vi "VCS Read Channel Data Vector.vi"(0 "axis in":cluster{"keyHandle":u32, "nodeId":u16}={"keyHandle"=0, "nodeId"=1}, 5 "channelNumber":u8, 7 "vectorSize":u32, 9 "objectSize":u8, 11 "error in (no error)":errorcluster) -> (4 "axis out":cluster{"keyHandle":u32, "nodeId":u16}={"keyHandle"=0, "nodeId"=1}, 8 "data vector":u8[](array[numeric]), 15 "error out":errorcluster)   [LabVIEW 2018]
doc: "<B>VCS_ReadChannelDataVector</B> returns the data points of a selected channel."
uses:
  Resources/EposCmd.dll
  Resources/EposCmd64.dll
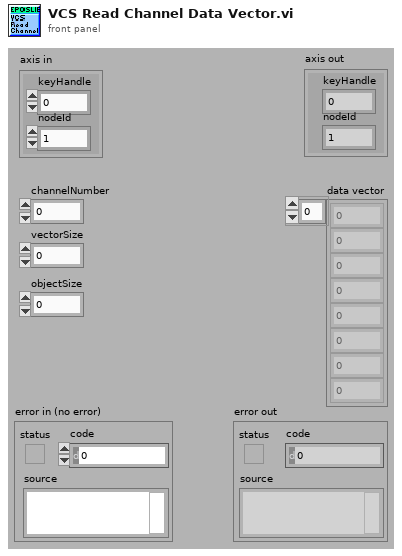
[diagram p1: front panel]
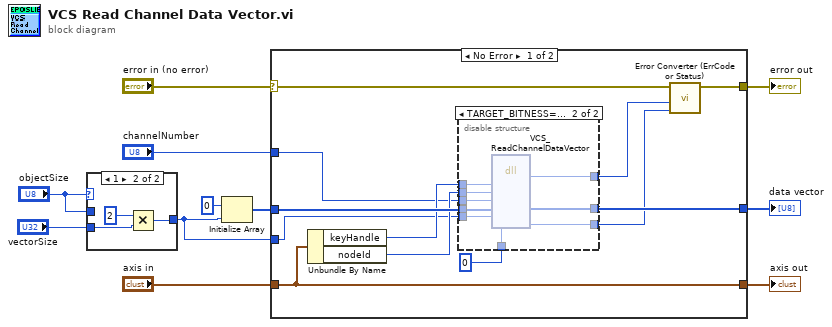
[diagram p0: block diagram]
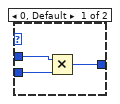
[diagram p2: hidden frame]
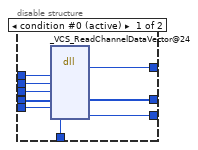
[diagram p3: hidden frame]
diagram:
  n1 = case shown="1" "objectSize" {
    tunnel: "vectorSize" -> [w13 w17]
    tunnel: "objectSize" -> [w14 _]
    tunnel: [w12 w15] -> w1
    frame 0, Default {
      n2 = Multiply(x=w14, y=w13) -> (x*y=w12:u32)
    }
    frame 1 {
      n3 = Multiply(x=u32 2, y=w17) -> (x*y=w15:u32)
    }
  }
  n4 = Initialize Array(u8 0, w1) -> (w6:u8[])
  n5 = case shown="No Error" "error in (no error)" {
    selector: "error in (no error)" -> [w27 w49]
    tunnel: "axis in" -> [w29 w50]
    tunnel: [w29 w50] -> w10
    tunnel: [w28 w49] -> w9
    tunnel: w6 -> [w26 w48]
    tunnel: [w25 w48] -> w5
    tunnel: "channelNumber" -> [w22 _]
    tunnel: w1 -> [w18 _]
    frame No Error {
      n6 = Unbundle By Name(w29) -> ("keyHandle"=w24:u32, "nodeId"=w23:u16)
      n7 = disable-structure shown="TARGET_BITNESS==64" {
        disable-tunnel: w26 -> [w38 w47]
        disable-tunnel: [w37 w46] -> w25
        disable-tunnel: w24 -> [w36 w45]
        disable-tunnel: w23 -> [w35 w44]
        disable-tunnel: w22 -> [w34 w43]
        disable-tunnel: u32 0 ("pErrorCode") -> [w33 w42]
        disable-tunnel: [w32 w41] -> w20
        disable-tunnel: [w31 w40] -> w19
        disable-tunnel: w18 -> [w30 w39]
        frame condition #0 (active) {
          n8 = dll-call lib="C:/Projeto em LabVIEW/EPOS-LabVIEW-Instrument-Driver-En/LabVIEW/maxon EPOS/Resources/EposCmd.*" fn="_VCS_ReadChannelDataVector@24" ("VCS_ReadChannelDataVector")("KeyHandle"=w36, "NodeId"=w35, "ChannelNumber"=w34, "pDataVector"=w38, "VectorSize"=w30, "pErrorCode"=w33) -> ("Rückgabetyp"=w31:i32, "pDataVector"=w37:u8[], "pErrorCode"=w32:u32)  [unwired: 7 in, 2 out]
        }
        frame condition #1 {
          n9 = dll-call lib="C:/setup/Resources/EposCmd64.*" fn="VCS_ReadChannelDataVector"("KeyHandle"=w45, "NodeId"=w44, "ChannelNumber"=w43, "pDataVector"=w47, "VectorSize"=w39, "pErrorCode"=w42) -> ("Rückgabetyp"=w40:i32, "pDataVector"=w46:u8[], "pErrorCode"=w41:u32)  [unwired: 7 in, 2 out]
        }
      }
      n10 = call "Error Converter (ErrCode or Status).vi"("error code"=w20, "return type"=w19, "error in (no error)"=w27) -> ("error out"=w28:errorcluster)  [unwired: 7 in]
    }
    frame Error {
    }
  }
  "data vector" <- w5
  "error out" <- w9
  "axis out" <- w10
